vi "jsTest.vi"() -> ()   [LabVIEW 2014]
panel:
  out "Array 2":string[](array[string])
  out "Array":dbl[](array[numeric])
  out "error out":errorcluster
  in  "stop":bool
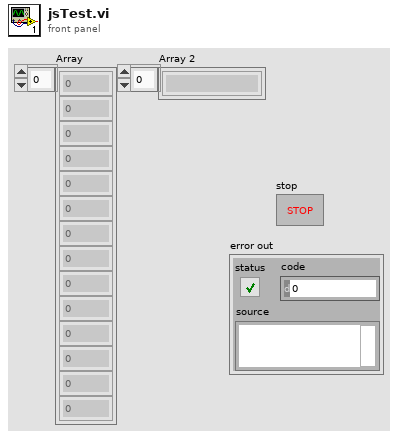
[diagram p1: front panel]
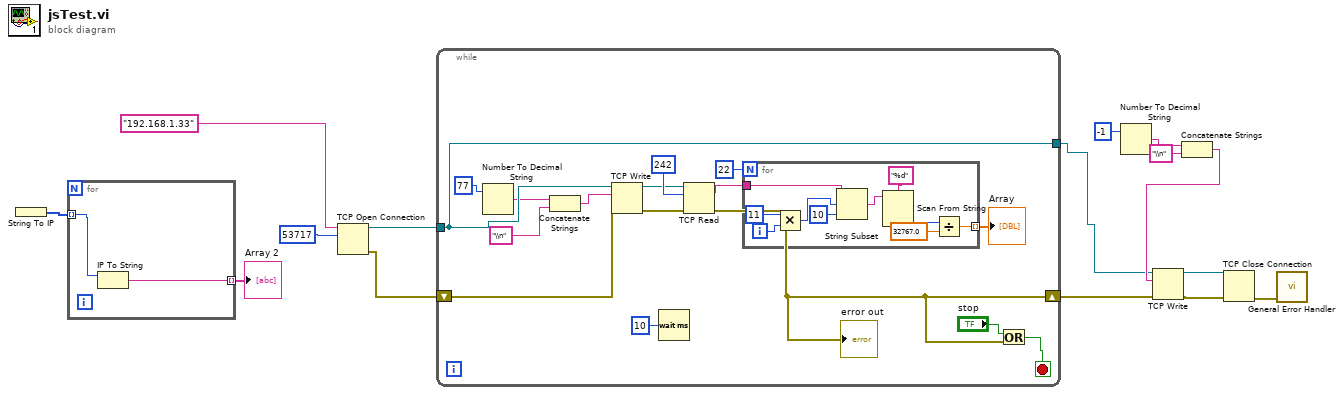
[diagram p0: block diagram]
diagram:
  n1 = String To IP() -> (0:w2:u32[])  [unwired: 1 in]
  n2 = for {
    tunnel: w2 -> [w17] mode=indexing
    tunnel: [w16] -> w1 mode=indexing
    n3 = IP To String(2:w17) -> (0:w16:string)  [unwired: 1 in]
  }
  "Array 2" <- w1
  n4 = TCP Open Connection(address="192.168.1.33", remote port or service name=u16 53717) -> (connection ID=w13:refnum<k5>, error out=w12:errorcluster)  [unwired: 3 in]
  n5 = while {
    tunnel: w13 -> [w29]
    tunnel: [w29] -> w5
    shift-right: [w25] -> w6
    shift-left: w12 -> [w30]
    stop <- w26 stop-if-true
    n6 = Number To Decimal String(number=77) -> (decimal integer string=w23:string)  [unwired: 1 in]
    n7 = Concatenate Strings(w23, "\\n" ("string")) -> (w21:string)
    n8 = TCP Write(connection ID=w29, data in=w21, error in (no error)=w30) -> (connection ID out=w32:refnum<k5>, error out=w31:errorcluster)  [unwired: 1 in, 1 out]
    n9 = Wait (ms)(milliseconds to wait=u32 10) -> ()  [unwired: 1 out]
    n10 = TCP Read(connection ID=w32, bytes to read=242, error in (no error)=w31) -> (data out=w18:string, error out=w25:errorcluster)  [unwired: 2 in, 1 out]
    "error out" <- w25
    n11 = for {
      N: 22 -> [_]
      tunnel: w18 -> [w43]
      tunnel: [w35] -> w19 mode=indexing
      i -> [w41]
      n12 = Multiply(x=11, y=w41) -> (x*y=w39:i32)
      n13 = String Subset(string=w43, offset (0)=w39, length (rest)=10 ("length (rest)")) -> (substring=w38:string)
      n14 = Scan From String(format string="%d", input string=w38) -> (output 1=w34:i32)  [unwired: 3 in, 3 out]
      n15 = Divide(x=w34, y=32767.0) -> (x/y=w35:dbl)
    }
    "Array" <- w19
    n16 = Or(x="stop", y=w25) -> (x .or. y?=w26:bool)
  }
  n17 = Number To Decimal String(number=-1) -> (decimal integer string=w9:string)  [unwired: 1 in]
  n18 = Concatenate Strings(w9, "\\n" ("string")) -> (w7:string)
  n19 = TCP Write(connection ID=w5, data in=w7, error in (no error)=w6) -> (connection ID out=w3:refnum<k5>, error out=w4:errorcluster)  [unwired: 1 in, 1 out]
  n20 = TCP Close Connection(connection ID=w3, error in (no error)=w4) -> (error out=w11:errorcluster)  [unwired: 1 in, 1 out]
  n21 = call <vilib>:"General Error Handler.vi"("error in (no error)"=w11) -> ()  [unwired: 10 in, 5 out]
